vi "Generate Pin Map Client.vi"() -> ()   [LabVIEW 2020]
panel:
  out "error out":errorcluster
  in  "error in (no error)":errorcluster
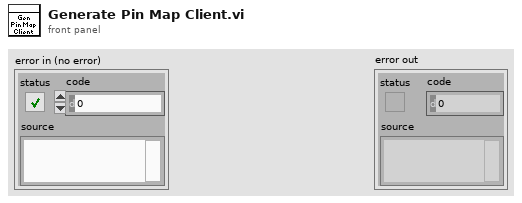
[diagram p1: front panel]
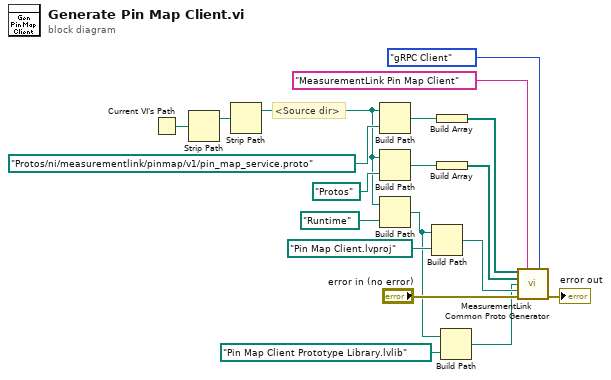
[diagram p0: block diagram]
diagram:
  # "<Source dir>"
  n1 = Current VI's Path() -> (path=w14:path)
  n2 = Strip Path(path=w14) -> (stripped path=w13:path)  [unwired: 1 out]
  n3 = Strip Path(path=w13) -> (stripped path=w15:path)  [unwired: 1 out]
  n4 = Build Path(base path=w15, name or relative path=path "Protos/ni/measurementlink/pinmap/v1/pin_map_service.proto" ("Proto File Path")) -> (appended path=w18:path)
  n5 = Build Path(base path=w15, name or relative path=path "Protos" ("Proto File Path")) -> (appended path=w16:path)
  n6 = Build Path(base path=w15, name or relative path=path "Runtime" ("Target Project")) -> (appended path=w3:path)
  n7 = Build Path(base path=w3, name or relative path=path "Pin Map Client.lvproj" ("Target Project")) -> (appended path=w4:path)
  n8 = Build Array(w18) -> (w6:path[])
  n9 = Build Array(w16) -> (w7:path[])
  n10 = Build Path(base path=w3, name or relative path=path "Pin Map Client Prototype Library.lvlib") -> (appended path=w1:path)
  n11 = call "MeasurementLink Common Proto Generator.vi"("Proto File Path"=w6, "Generated Library Full Name"="MeasurementLink Pin Map Client" ("Generated Library Name"), "Generate"=enum16{"gRPC Server", "gRPC Client", "Both"}."gRPC Client", "Import Paths"=w7, "Prototype Library"=w1, "Target Project"=w4, "error in (no error)"="error in (no error)") -> ("error out"=→"error out":errorcluster)  [unwired: 8 in]
